vi "Calc Go to SP.vi"(7 "Direction":T1=enum."DUT", 8 "error in (no error)":errorcluster, 11 "Stand in":refnum<class "Stand.lvclass">) -> (0 "error out":errorcluster, 3 "Stand out":refnum<class "Stand.lvclass">)   [LabVIEW 2019, in "Stand.lvclass"]
uses:
  Stand.lvclass
  TypeDef/Direction.ctl
  Stand.lvclass/Stand.ctl
  AI_class/AI.lvclass/AI.ctl
  AnalogComparator_class/AnalogComparator.lvclass/AnalogComparator.ctl
  OscillationClass/OscillationDetector.lvclass/OscillationDetector.ctl
  TypeDef/ScriptName.ctl
  AnalogComparator_class/GetStatus.vi
  OscillationClass/Read DATA.vi
  AI_class/AI.lvclass
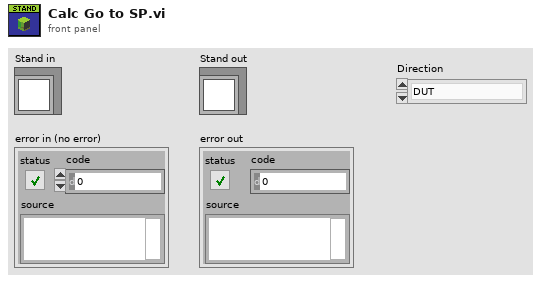
[diagram p1: front panel]
types:
  T1 = typedef "Direction.ctl" = enum16{"None", "DUT", "Chamber"}
  T2 = typedef "ScriptName.ctl" = enum16{"Alarm", "Filling DUT", "Filling Chamber", "Measure Haskel T0 DUT", "Measure Haskel T0 Chamber", "Measure Pump T0 DUT", "Measure Pump T0 Chamber", "Low Pressure DUT", "Low Pressure Chamber", "Hi Pressure Dut", "Hi Pressure Chamber", "Stop Pump", "HaskelFastForward DUT", "HaskelFastForward Chamber", "PumpFastForward DUT", "PumpFastForward Chamber", "Pressure Realise DUT", "Pressure Realise Chamber"}
  T3 = typedef "AI_Data.ctl" = cluster{"Stat Data":T4, "OutOfRangeMax":bool, "OutOfRangeMin":bool, "HIHI":bool, "HI":bool, "LO":bool, "LOLO":bool, "DATA N":T5, "DATA PERIOD":T5, "UPPER TH":dbl, "LOWER TH":dbl}
  T4 = typedef "AI Statistics Data.ctl" = cluster{"raw mean":dbl, "scl mean":dbl, "raw mean 1Hz":dbl, "scl mean 1Hz":dbl}
  T5 = typedef "DATA Oscill.ctl" = cluster{"SUM":dbl, "COUNTER":dbl, "MAX CURR":dbl, "MIN CURR":dbl, "AVR":dbl, "MAX":dbl, "MIN":dbl, "DELTA AVR":dbl, "DELTA MAX":dbl, "DELTA MIN":dbl, "PERIOD":dbl}
  T6 = typedef "Action.ctl" = enum16{"Air: On", "Air: Off", "Pump Station: On (Filling Mode)", "Pump Station: On (Pressure Mode)", "Pump Station: Off", "Air Valves: Open (DUT Filling)", "Air Valves: Open (Chamber Filling)", "Air Valves: Open (Pump Pressure DUT)", "Air Valves: Open (Pump Pressure Chamber)", "Air Valves: Open (Haskel Pressure DUT)", "Air Valves: Open (Haskel Pressure Chamber)", "Air Valves: Open (Slow Release DUT)", "Air Valves: Open (Slow Release Chamber)", "Air Valves: Open (Fast Release DUT)", "Air Valves: Open (Fast Release Chamber)", "Air Valves: Open (Emergency Release DUT and Chamber)", "Air Valves: Open (Leak Test Pressure Sensor 41.3)", "Air Valves: Open (Leak Test Burette 42)", "Air Valves: Fully Closed", "Haskel: Off (0)", "Haskel: Pressure Control (PI Regulator) DUT", "Haskel: Pressure Control (PI Regulator) Chamber", "Haskel: Measure T0 DUT", "Haskel: Measure T0 Chamber", "Haskel: FastForward DUT", "Haskel: FastForward Chamber", "Proportional Valve: Off (0)", "Proportional Valve: Pressure Control (PI Regulator) DUT", "Proportional Valve: Pressure Control (PI Regulator) Chamber", "Proportional Valve: Measure T0 DUT", "Proportional Valve: Measure T0 Chamber", "Proportional Valve: FastForward DUT", "Proportional Valve: FastForward Chamber", "Valve 44.1: Open", "Valve 44.1: Close", "Valve 44.2: Open", "Valve 44.2: Close", "Valve 37.1: Open", "Valve 37.1: Close", "Valve 37.2: Open", "Valve 37.2: Close", "Filling: In Progress DUT", "Filling: In Progress Chamber", "Pressure pre loading: DUT", "Pressure pre loading: Chamber", "Slow Pressure Release: In Progress (DUT)", "Slow Pressure Release: In Progress (Chamber)", "NONE"}
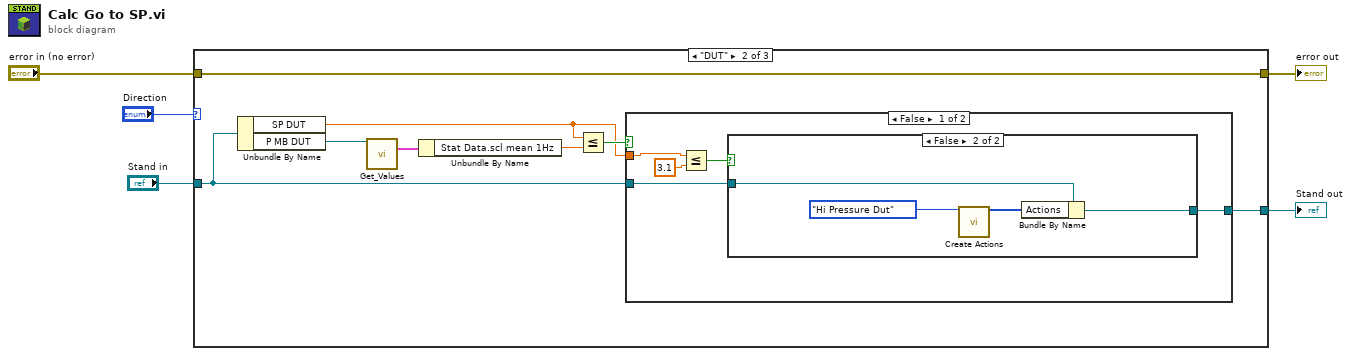
[diagram p0: block diagram]
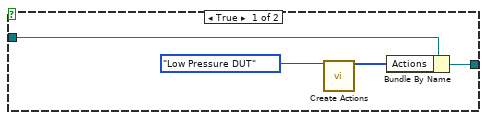
[diagram p3: hidden frame]
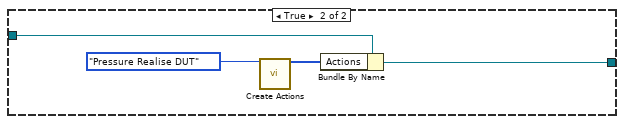
[diagram p4: hidden frame]
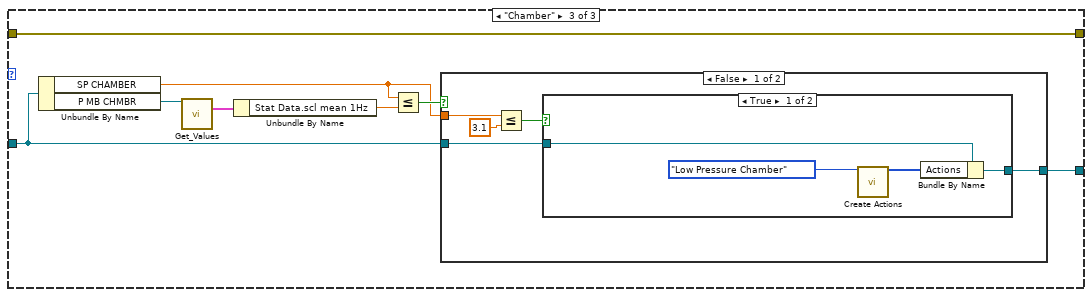
[diagram p5: hidden frame]
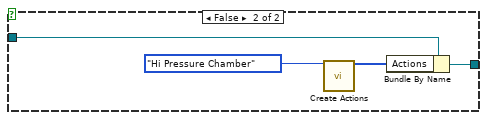
[diagram p6: hidden frame]
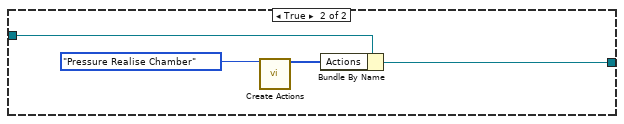
[diagram p7: hidden frame]
diagram:
  n1 = case shown="\"DUT\"" "Direction" {
    tunnel: "error in (no error)" -> [w6 w9 w34]
    tunnel: "Stand in" -> [w7 w10 w35]
    tunnel: [w7 w11 w36] -> w2
    tunnel: [w6 w9 w34] -> w1
    frame "None" {
    }
    frame "DUT" {
      n2 = Unbundle By Name(w10) -> ("SP DUT"=w8:dbl, "P MB DUT"=w15:refnum<class "AI.lvclass">)
      n3 = call "Get_Values.vi"("reference in"=w15) -> ("Data"=w14:T3)  [unwired: 14 in]
      n4 = Unbundle By Name(w14) -> ("Stat Data.scl mean 1Hz"=w13:dbl)
      n5 = Less Or Equal?(x=w8, y=w13) -> (x <= y?=w12:bool)
      n6 = case shown="False" w12 {
        tunnel: [w16 w30] -> w11
        tunnel: w10 -> [w17 w32]
        tunnel: w8 -> [w20 _]
        frame False {
          n7 = Less Or Equal?(x=w20, y=3.1) -> (x <= y?=w18:bool)
          n8 = case shown="False" w18 {
            tunnel: w17 -> [w22 w26]
            tunnel: [w21 w25] -> w16
            frame True {
              n9 = call "Create Actions.vi"("Script"=ScriptName."Low Pressure DUT") -> ("Actions out"=w24:T6[])  [unwired: 14 in]
              n10 = Bundle By Name(cluster=w22, "Actions"=w24) -> (w21:refnum<class "Stand.lvclass">)
            }
            frame False {
              n11 = call "Create Actions.vi"("Script"=ScriptName."Hi Pressure Dut") -> ("Actions out"=w28:T6[])  [unwired: 14 in]
              n12 = Bundle By Name(cluster=w26, "Actions"=w28) -> (w25:refnum<class "Stand.lvclass">)
            }
          }
        }
        frame True {
          n13 = call "Create Actions.vi"("Script"=ScriptName."Pressure Realise DUT") -> ("Actions out"=w29:T6[])  [unwired: 14 in]
          n14 = Bundle By Name(cluster=w32, "Actions"=w29) -> (w30:refnum<class "Stand.lvclass">)
        }
      }
    }
    frame "Chamber" {
      n15 = Unbundle By Name(w35) -> ("SP CHAMBER"=w33:dbl, "P MB CHMBR"=w40:refnum<class "AI.lvclass">)
      n16 = call "Get_Values.vi"("reference in"=w40) -> ("Data"=w39:T3)  [unwired: 14 in]
      n17 = Unbundle By Name(w39) -> ("Stat Data.scl mean 1Hz"=w38:dbl)
      n18 = Less Or Equal?(x=w33, y=w38) -> (x <= y?=w37:bool)
      n19 = case shown="False" w37 {
        tunnel: [w41 w55] -> w36
        tunnel: w35 -> [w42 w57]
        tunnel: w33 -> [w45 _]
        frame False {
          n20 = Less Or Equal?(x=w45, y=3.1) -> (x <= y?=w43:bool)
          n21 = case shown="True" w43 {
            tunnel: w42 -> [w47 w51]
            tunnel: [w46 w50] -> w41
            frame True {
              n22 = call "Create Actions.vi"("Script"=ScriptName."Low Pressure Chamber") -> ("Actions out"=w49:T6[])  [unwired: 14 in]
              n23 = Bundle By Name(cluster=w47, "Actions"=w49) -> (w46:refnum<class "Stand.lvclass">)
            }
            frame False {
              n24 = call "Create Actions.vi"("Script"=ScriptName."Hi Pressure Chamber") -> ("Actions out"=w53:T6[])  [unwired: 14 in]
              n25 = Bundle By Name(cluster=w51, "Actions"=w53) -> (w50:refnum<class "Stand.lvclass">)
            }
          }
        }
        frame True {
          n26 = call "Create Actions.vi"("Script"=ScriptName."Pressure Realise Chamber") -> ("Actions out"=w54:T6[])  [unwired: 14 in]
          n27 = Bundle By Name(cluster=w57, "Actions"=w54) -> (w55:refnum<class "Stand.lvclass">)
        }
      }
    }
  }
  "Stand out" <- w2
  "error out" <- w1
